vi "testFlattenMassToXML.vi"() -> ()   [LabVIEW 2012, in "UnitsAndXML.lvlib"]
uses:
  <userlib>/Common/UnitsAndXML/UnitsAndXML.lvlib
  <userlib>/Common/UnitsAndXML/FlattenItemWithUnitToXML/FlattenMassToXML/MassUnit.ctl
  <userlib>/Common/UnitsAndXML/FlattenItemWithUnitToXML/FlattenMassToXML/typeMethods/flattenMassToXML_Array.vi
  <userlib>/Common/UnitsAndXML/FlattenItemWithUnitToXML/FlattenMassToXML/typeMethods/flattenMassToXML_Scalar.vi
panel:
  out "error out":errorcluster
  in  "massUnitInXML":T1
  out "xmlStringArray":string
  out "xmlStringScalar":string
  in  "mass":dbl[unit][](array[numeric])=[6.8038855499999995, 13.607771099999999, 20.41165665, 27.215542199999998]
  in  "mass":dbl[unit]=6.8038855499999995
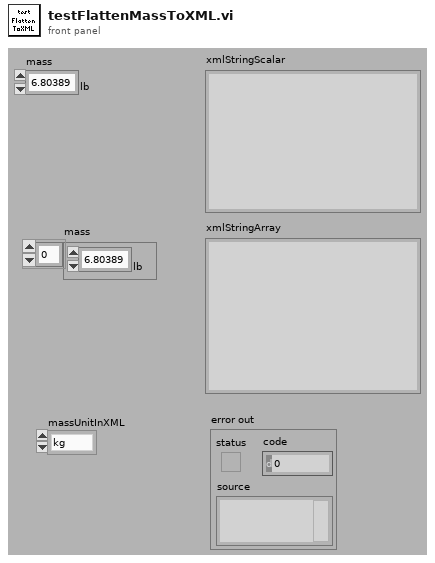
[diagram p1: front panel]
types:
  T1 = typedef "UnitsAndXML.lvlib/MassUnit.ctl" = enum16{"kg", "CM", "dr", "gr", "t", "oz", "lb", "slug", "stone", "Ton", "ton", "u"}
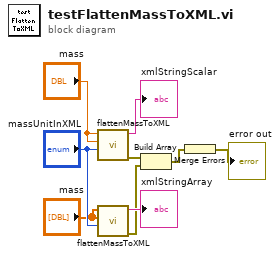
[diagram p0: block diagram]
diagram:
  n1 = call-poly <userlib>:"flattenMassToXML.vi"("massUnitInXML"="massUnitInXML", "massAgain"="mass", "mass"="mass") -> ("error out"=w6:errorcluster, "xmlString"=→"xmlStringScalar":string)  [unwired: 7 in]
  n2 = call-poly <userlib>:"flattenMassToXML.vi"("massUnitInXML"="massUnitInXML", "massAgain"="mass", "mass"="mass") -> ("error out"=w1:errorcluster, "xmlString"=→"xmlStringArray":string)  [unwired: 7 in]
  n3 = Build Array(w6, w1) -> (w7:errorcluster[])
  n4 = Merge Errors(w7) -> (→"error out":errorcluster)
